vi "Cluster Generate Datatype Name.vi"(10 "Cluster elements names":string[](array[string]), 11 "Cluster elements datatypes":string[](array[string])) -> (3 "generated datatype name":string)   [LabVIEW 2014]
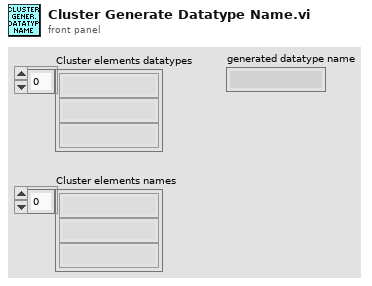
[diagram p1: front panel]
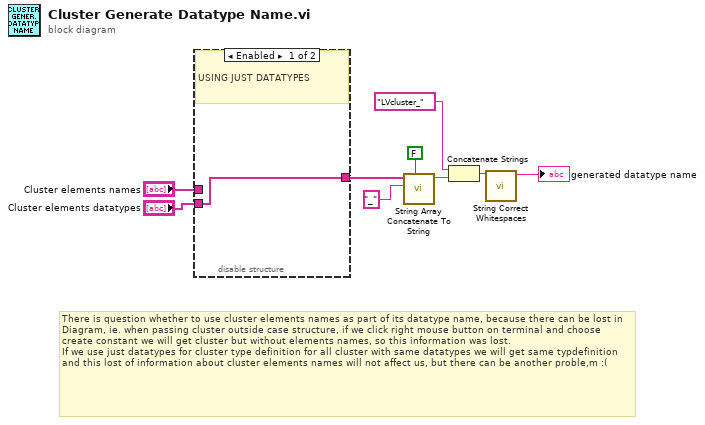
[diagram p0: block diagram]
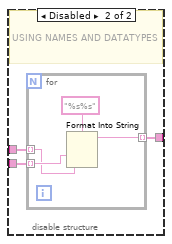
[diagram p2: hidden frame]
diagram:
  # "There is question whether to use cluster elements names as part of its datatype name, because there can be lost in Diagram, ie. when passing cluster outside case structure, if we click right mouse button on terminal and choose create constant we will get cluster but without elements names, so this information was lost.\nIf we use just datatypes for cluster type definition for all cluster with same datatypes we will get same typdefinition and this lost of information about cluster elements names will not affect us, but there can be another proble,m :("
  n1 = disable-structure shown="Enabled" {
    disable-tunnel: "Cluster elements datatypes" -> [w10 w13]
    disable-tunnel: "Cluster elements names" -> [_ w12]
    disable-tunnel: [w10 w11] -> w5
    frame Enabled {
      # "USING JUST DATATYPES"
    }
    frame Disabled {
      # "USING NAMES AND DATATYPES"
      n2 = for {
        tunnel: w13 -> [w15] mode=indexing
        tunnel: w12 -> [w14] mode=indexing
        tunnel: [w16] -> w11 mode=indexing
        n3 = Format Into String(format string="%s%s", w15, w14) -> (resulting string=w16:string)  [unwired: 2 in, 1 out]
      }
    }
  }
  n4 = call "String Array Concatenate To String.vi"("insert last delimiter?"=FALSE, "Delimiter char"="_", "Array String In"=w5) -> ("String"=w4:string)  [unwired: 8 in]
  n5 = Concatenate Strings("LVcluster_" ("format string"), w4) -> (w2:string)
  n6 = call "String Correct Whitespaces.vi"("String in"=w2) -> ("String out"=→"generated datatype name":string)  [unwired: 10 in]
